vi "创建数据表.vi"(8 "error in (no error)":errorcluster) -> (0 "error out":errorcluster)   [LabVIEW 2016, in "数据查询.lvlib"]
uses:
  <vilib>/addons/database/Auxilliary.llb/DB Tools Column Info.ctl
  <vilib>/addons/database/Auxilliary.llb/DB Tools DataTypes.ctl
  <vilib>/addons/database/Connection.llb/DB Tools Open Connec (String).vi
  <userlib>/_LVST/sqlite_api/Core/Tables/SQLite_Drop Table.vi
  <userlib>/_LVST/sqlite_api/Core/Tables/SQLite_Create Table.vi
  <vilib>/addons/database/NI_Database_API.lvlib
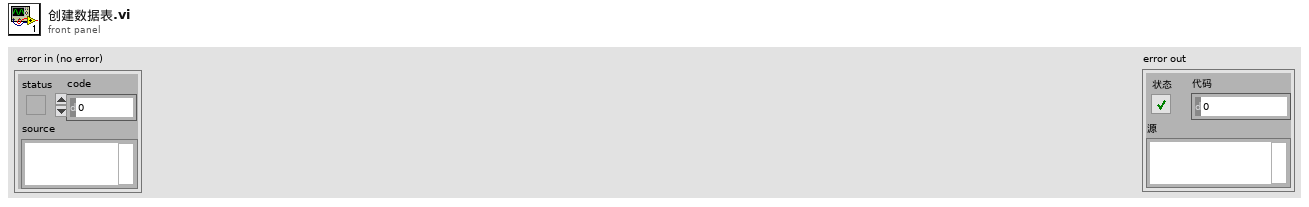
[diagram p1: front panel]
types:
  T1 = typedef "数据库类型.ctl" = enum16{"Access", "SQLite"}
  T2 = typedef "NI_Database_API.lvlib/DB Tools Column Info.ctl" = cluster{"column name":string, "data type":T3, "size":i32, "allow null?":bool}
  T3 = typedef "NI_Database_API.lvlib/DB Tools DataTypes.ctl" = enum16{"String", "Long (I32)", "Single (SGL)", "Double (DBL)", "Date/Time", "Binary"}
  T4 = typedef "NI_Database_API.lvlib/Conn ObjectReference.ctl" = refnum<k1>
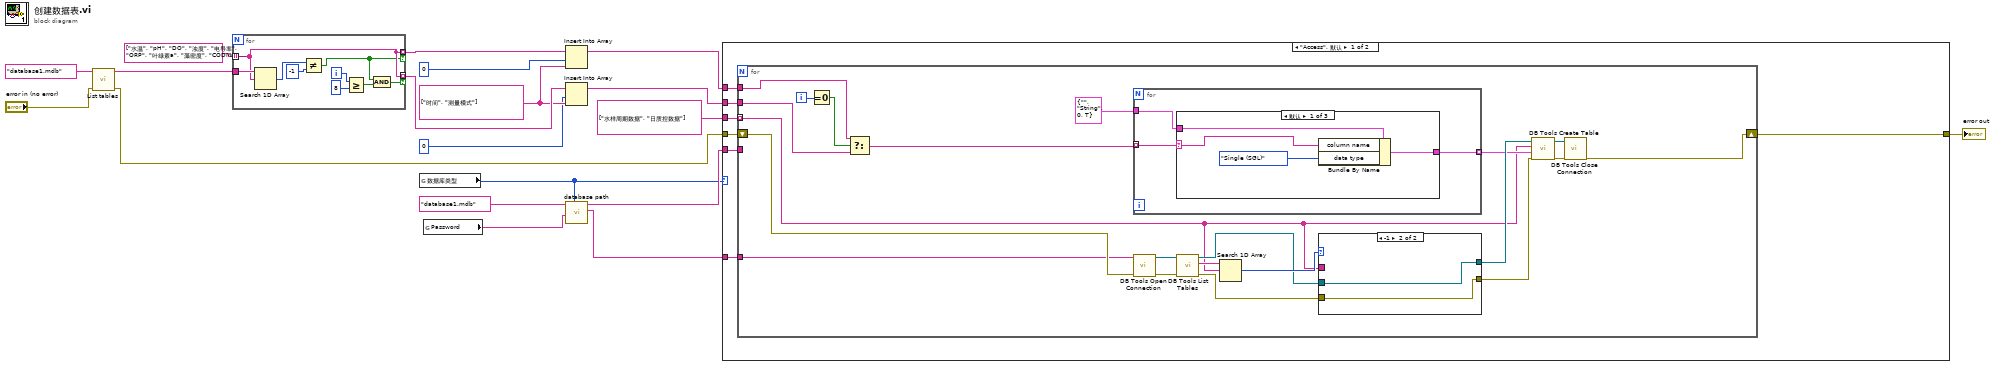
[diagram p0: block diagram]
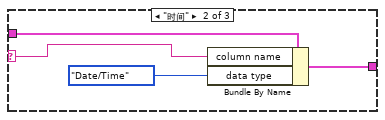
[diagram p2: hidden frame]
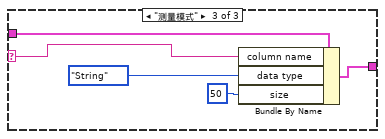
[diagram p3: hidden frame]
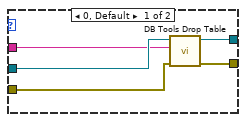
[diagram p4: hidden frame]
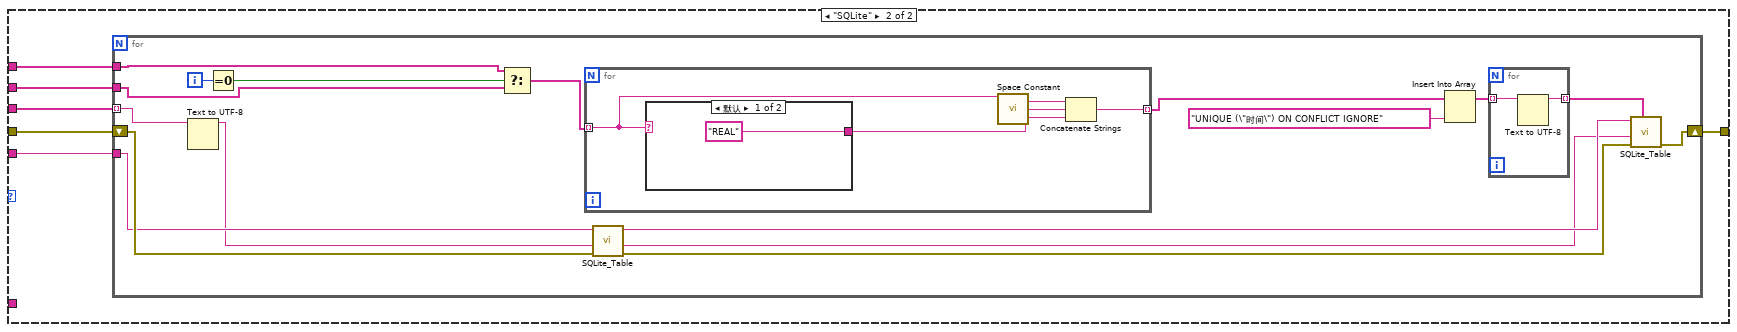
[diagram p5: hidden frame]
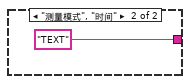
[diagram p6: hidden frame]
diagram:
  w14 = string[] ["时间", "测量模式"]
  n1 = call "List tables.vi"("error in (no error)"="error in (no error)", "database"="database1.mdb") -> ("error out"=w11:errorcluster, "tables"=w19:string[])  [unwired: 8 in]
  n2 = for {
    tunnel: string[] ["水温", "pH", "DO", "浊度", "电导率", "ORP", "叶绿素a", "藻密度", "CODMn", "CODcr", "COD", "磷酸盐", "氨氮", "总磷", "总氮", "亚硝氮", "硫化物", "硝氮", "硅酸盐"] -> [w25] mode=indexing
    tunnel: w19 -> [w28]
    tunnel: [w25] -> w18 mode=indexing if=w20
    tunnel: [w25] -> w15 mode=indexing if=w21
    i -> [w24]
    n3 = Search 1D Array(1D array=w28, element=w25) -> (index of element=w27:i32)  [unwired: 1 in]
    n4 = Not Equal?(x=w27, y=-1 ("x")) -> (x != y?=w20:bool)
    n5 = Greater Or Equal?(x=w24, y=8) -> (x >= y?=w22:bool)
    n6 = And(x=w20, y=w22) -> (x .and. y?=w21:bool)
  }
  n7 = global read "全局变量.vi" "数据库类型"() -> (w3:T1)
  n8 = global read "全局变量.vi" "Password"() -> (w1:string)
  n9 = Insert Into Array(array=w18, index=0 ("索引"), new element=w14) -> (w10:string[])
  n10 = Insert Into Array(array=w15, index=0 ("索引"), new element=w14) -> (w8:string[])
  n11 = call "database path.vi"("数据库类型"=w3, "Password"=w1, "database"="database1.mdb") -> ("Connection information"=w2:string, "Path out"=w4:string)  [unwired: 7 in]
  n12 = case shown="\"Access\", 默认" w3 {
    tunnel: w10 -> [w35 w84]
    tunnel: w11 -> [w34 w81]
    tunnel: [w33 w82] -> w6
    tunnel: string[] ["水样周期数据", "日质控数据"] -> [w32 w85]
    tunnel: w8 -> [w31 w83]
    tunnel: w4 -> [w30 w80]
    tunnel: w2 -> [w29 _]
    frame "Access", Default {
      n13 = for {
        tunnel: w35 -> [w39]
        shift-right: [w43] -> w33
        shift-left: w34 -> [w44]
        tunnel: w32 -> [w42] mode=indexing
        tunnel: w31 -> [w38]
        tunnel: w30 -> [_]
        tunnel: w29 -> [w36]
        i -> [w41]
        n14 = Equal To 0?(x=w41) -> (x = 0?=w40:bool)
        n15 = Select(t=w39, s=w40, f=w38) -> (s? t:f=w37:string[])
        n16 = for {
          tunnel: w37 -> [w59] mode=indexing
          tunnel: T2 {"column name"="", "data type"=enum."String", "size"=0, "allow null?"=TRUE} ("column information") -> [w58]
          tunnel: [w57] -> w45 mode=indexing
          n17 = case shown="默认" w59 {
            selector: w59 -> [w62 w66 w71]
            tunnel: w58 -> [w63 w67 w72]
            tunnel: [w61 w65 w70] -> w57
            frame Default {
              n18 = Bundle By Name(cluster=w63, "column name"=w62, "data type"=DB_Tools_DataTypes."Single (SGL)") -> (w61:T2)
            }
            frame "时间" {
              n19 = Bundle By Name(cluster=w67, "column name"=w66, "data type"=DB_Tools_DataTypes."Date/Time") -> (w65:T2)
            }
            frame "测量模式" {
              n20 = Bundle By Name(cluster=w72, "column name"=w71, "data type"=DB_Tools_DataTypes."String", "size"=50) -> (w70:T2)
            }
          }
        }
        n21 = call-poly <vilib>:"DB Tools Open Connection.vi"("error in (no error)"=w44, "connection information"=w36) -> ("error out"=w56:errorcluster, "connection reference"=w55:T4)  [unwired: 6 in]
        n22 = call <vilib>:"DB Tools List Tables.vi"("error in (no error)"=w56, "connection reference"=w55) -> ("error out"=w50:errorcluster, "tables"=w54:string[], "connection reference out"=w52:T4)  [unwired: 3 in]
        n23 = Search 1D Array(1D array=w54, element=w42) -> (index of element=w53:i32)  [unwired: 1 in]
        n24 = case shown="-1" w53 {
          tunnel: w52 -> [w77 w79]
          tunnel: [w76 w79] -> w51
          tunnel: w50 -> [w75 w78]
          tunnel: [w74 w78] -> w49
          tunnel: w42 -> [w73 _]
          frame 0, Default {
            n25 = call <vilib>:"DB Tools Drop Table.vi"("error in (no error)"=w75, "table"=w73, "connection reference"=w77) -> ("error out"=w74:errorcluster, "connection reference out"=w76:T4)  [unwired: 5 in]
          }
          frame -1 {
          }
        }
        n26 = call <vilib>:"DB Tools Create Table.vi"("error in (no error)"=w49, "column information"=w45, "table"=w42, "connection reference"=w51) -> ("error out"=w47:errorcluster, "connection reference out"=w48:T4)  [unwired: 4 in]
        n27 = call <vilib>:"DB Tools Close Connection.vi"("error in (no error)"=w47, "connection reference"=w48) -> ("error out"=w43:errorcluster)  [unwired: 5 in]
      }
    }
    frame "SQLite" {
      n28 = for {
        tunnel: w80 -> [w90]
        tunnel: w85 -> [w89] mode=indexing
        tunnel: w84 -> [w97]
        tunnel: w83 -> [w96]
        shift-right: [w94] -> w82
        shift-left: w81 -> [w93]
        i -> [w99]
        n29 = Text to UTF-8(11:w89) -> (3:w88:string)  [unwired: 2 in, 1 out]
        n30 = Equal To 0?(x=w99) -> (x = 0?=w98:bool)
        n31 = Select(t=w97, s=w98, f=w96) -> (s? t:f=w95:string[])
        n32 = for {
          tunnel: w95 -> [w108] mode=indexing
          tunnel: [w105] -> w91 mode=indexing
          n33 = case shown="默认" w108 {
            tunnel: ["REAL" "TEXT"] -> w106
            frame Default {
            }
            frame "测量模式", "时间" {
            }
          }
          n34 = call <vilib>:"Space Constant.vi"() -> ("String"=w107:string)
          n35 = Concatenate Strings(w108, w107, w106) -> (w105:string)
        }
        n36 = call-poly <userlib>:"SQLite_Table.vi"("DB Path"=w90, "Table Name"=w88, "error in (no error)"=w93) -> ("DB Path Out"=w102:string, "Table Name Out"=w100:string, "error out"=w101:errorcluster)  [unwired: 5 in]
        n37 = Insert Into Array(array=w91, new element="UNIQUE (\"时间\") ON CONFLICT IGNORE" ("新元素/子数组")) -> (w87:string[])  [unwired: 1 in]
        n38 = for {
          tunnel: w87 -> [w104] mode=indexing
          tunnel: [w103] -> w86 mode=indexing
          n39 = Text to UTF-8(11:w104) -> (3:w103:string)  [unwired: 2 in, 1 out]
        }
        n40 = call-poly <userlib>:"SQLite_Table.vi"("DB Path"=w102, "Table Name"=w100, "error in (no error)"=w101, "Columns"=w86) -> ("error out"=w94:errorcluster)  [unwired: 4 in, 2 out]
      }
    }
  }
  "error out" <- w6
